vi "ukol4.vi"(8 "dt":dbl, 11 "Y":dbl[](array[numeric])) -> (0 "Array 2":dbl[](array[numeric]), 1 "Array 3":bool[](array[boolean]), 2 "x/y 2":dbl[](array[numeric]), 3 "Array":dbl[](array[numeric]))   [LabVIEW 2023]
uses:
  <vilib>/measure/NI_MABase.lvlib
  <vilib>/Analysis/NI_AALPro.lvlib
panel:
  out "x/y":dbl[](array[numeric])
  out "Waveform Graph":waveform(dbl)(graph)
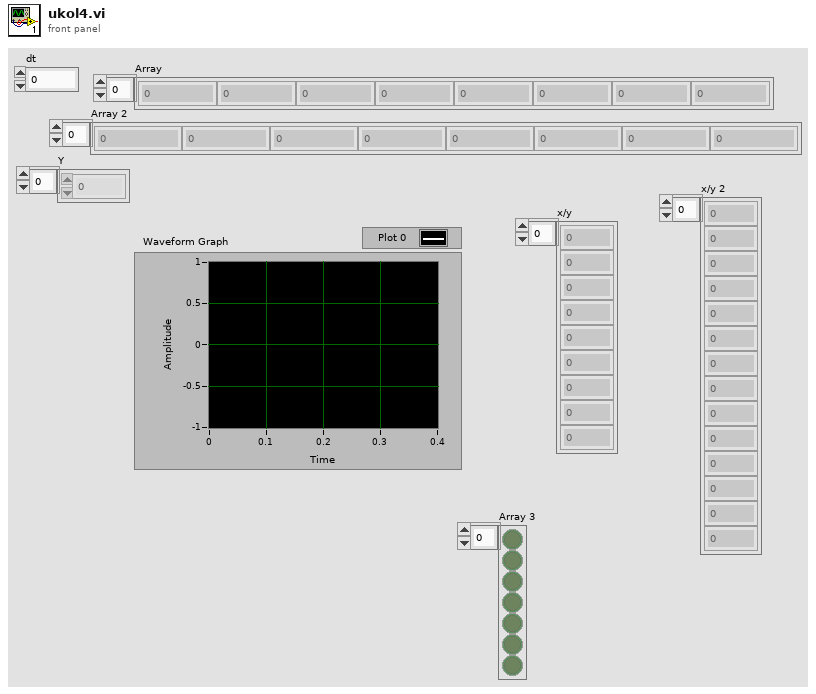
[diagram p1: front panel]
types:
  T1 = cluster{"frequency":dbl, "amplitude":dbl, "phase":dbl}[]
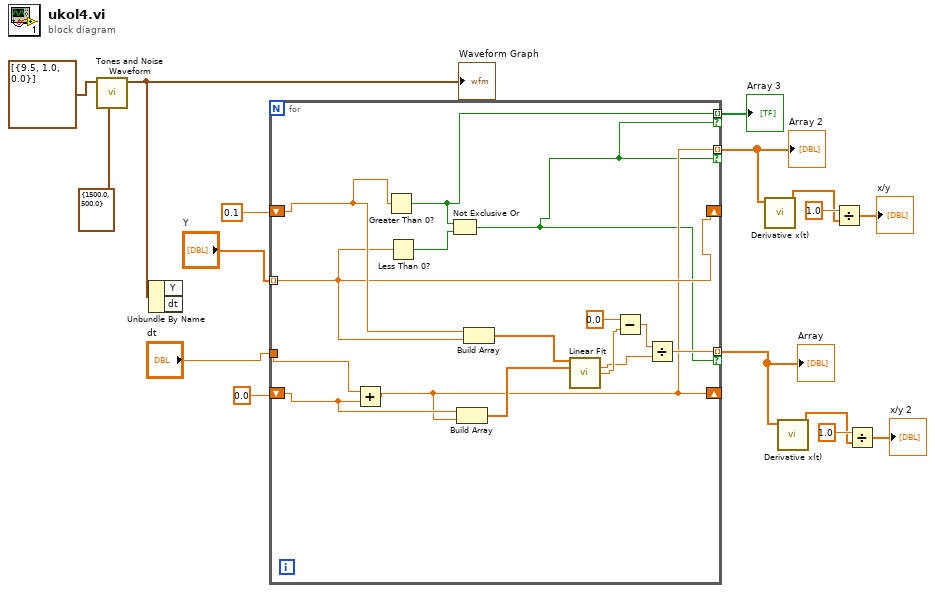
[diagram p0: block diagram]
diagram:
  n1 = call <vilib>:"Tones and Noise Waveform.vi"("sampling info"=cluster{"Fs":dbl, "#s":dbl} {"Fs"=1500.0, "#s"=500.0}, "tones"=T1 [{"frequency"=9.5, "amplitude"=1.0, "phase"=0.0}]) -> ("signal out"=w14:waveform(dbl))  [unwired: 8 in, 1 out]
  "Waveform Graph" <- w14
  n2 = Unbundle By Name(w14) -> ()  [unwired: 2 out]
  n3 = for {
    tunnel: "Y" -> [w22] mode=indexing
    shift-right: [w22] -> _
    shift-left: 0.1 -> [w23]
    tunnel: "dt" -> [w29]
    shift-right: [w19] -> _
    shift-left: 0.0 -> [w26]
    tunnel: [w27] -> w5 mode=indexing if=w17
    tunnel: [w19] -> w4 mode=indexing if=w17
    tunnel: [w18] -> w3 mode=indexing if=w17
    n4 = Add(x=w29, y=w26) -> (x+y=w19:dbl)
    n5 = Greater Than 0?(x=w23) -> (x > 0?=w18:bool)
    n6 = Less Than 0?(x=w22) -> (x < 0?=w31:bool)
    n7 = Not Exclusive Or(1:w31, 2:w18) -> (0:w17:bool)
    n8 = Build Array(w26, w19) -> (w28:dbl[])
    n9 = Build Array(w23, w22) -> (w30:dbl[])
    n10 = call <vilib>:"Linear Fit.vi"("Y"=w30, "X"=w28) -> ("slope"=w20:dbl, "intercept"=w21:dbl)  [unwired: 9 in, 3 out]
    n11 = Subtract(x=0.0, y=w21) -> (x-y=w25:dbl)
    n12 = Divide(x=w25, y=w20) -> (x/y=w27:dbl)
  }
  "Array" <- w5
  "Array 2" <- w4
  "Array 3" <- w3
  n13 = call <vilib>:"Derivative x(t).vi"("X"=w4) -> ("dX/dt"=w10:dbl[])  [unwired: 9 in, 1 out]
  n14 = call <vilib>:"Derivative x(t).vi"("X"=w5) -> ("dX/dt"=w7:dbl[])  [unwired: 9 in, 1 out]
  n15 = Divide(x=1.0, y=w10) -> (x/y=→"x/y":dbl[])
  n16 = Divide(x=1.0, y=w7) -> (x/y=→"x/y 2":dbl[])
